vi "Analysis.Process.vi"(8 "error in (no error)":errorcluster, 11 "Parameters":T1) -> ()   [LabVIEW 2015, in "Analysis.lvlib"]
uses:
  Analysis.lvlib
  Types/Analysis.GUI.Parameters.ctl
  <vilib>/NI/AMC/Read Termination Message.vi
  <vilib>/NI/AMC/Create Single Message.vi
  <vilib>/NI/AMC/Globals.vi
  <vilib>/NI/AMC/AMC.lvlib
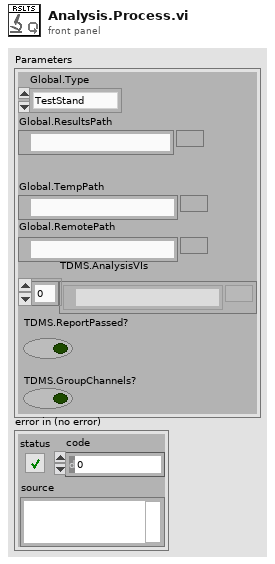
[diagram p1: front panel]
types:
  T1 = typedef "Analysis.lvlib/Analysis.GUI.Parameters.ctl" = cluster{"Global.Type":enum16{"TestStand", "TDMS"}, "Global.ResultsPath":path, "Global.TempPath":path, "Global.RemotePath":path, "TDMS.AnalysisVIs":path[], "TDMS.ReportPassed?":bool, "TDMS.GroupChannels?":bool}
  T2 = typedef "AMC.lvlib/Message Queue.ctl" = refnum<queue>
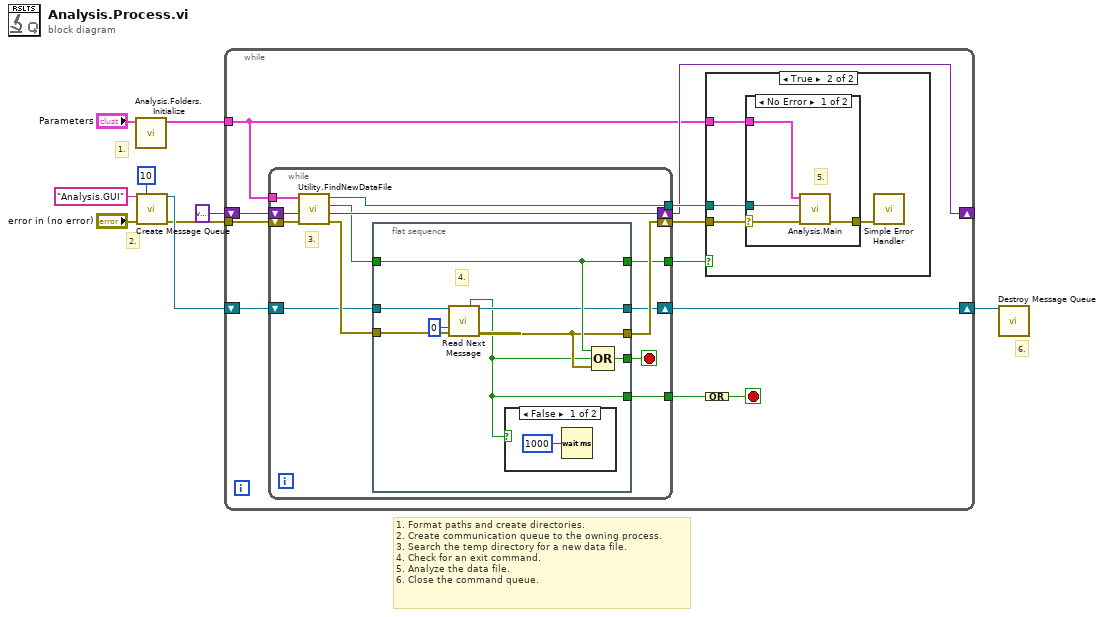
[diagram p0: block diagram]
diagram:
  # "6."
  # "1. Format paths and create directories.\n2. Create communication queue to the owning process.\n3. Search the temp directory for a new data file.\n4. Check for an exit command.\n5. Analyze the data file.\n6. Close the command queue."
  # "2."
  # "1."
  n1 = call "Analysis.Folders.Initialize.vi"("Parameters in"="Parameters") -> ("Parameters out"=w2:T1)  [unwired: 10 in]
  n2 = call <vilib>:"Create Message Queue.vi"("message queue name"="Analysis.GUI", "max queue size (-1, unlimited)"=10, "error in"="error in (no error)") -> ("message queue out"=w8:T2, "error out"=w7:errorcluster)  [unwired: 11 in]
  n3 = while {
    tunnel: w7 -> [w18]
    shift-right: [w15] -> _
    shift-left: variant -> [w16]
    tunnel: w2 -> [w12]
    shift-right: [w10] -> w9
    shift-left: w8 -> [w11]
    stop <- w19 stop-if-true
    n4 = while {
      shift-right: [w41] -> w14
      shift-left: w18 -> [w30]
      tunnel: [w34] -> w17
      tunnel: [w40] -> w13
      tunnel: [w38] -> w20
      shift-right: [w36] -> w15
      shift-left: w16 -> [w37]
      tunnel: w12 -> [w33]
      shift-right: [w31] -> w10
      shift-left: w11 -> [w32]
      stop <- w39 stop-if-true
      # "3."
      n5 = call "Utility.FindNewDataFile.vi"("error in (no error)"=w30, "LookupTable"=w37, "Parameters"=w33) -> ("error out"=w42:errorcluster, "LookupTable out"=w36:variant, "Found"=w35:bool, "Data Path"=w34:path)  [unwired: 5 in]
      n6 = flat-sequence {
        tunnel: w35 -> [w49]
        tunnel: [w50] -> w39
        tunnel: w42 -> [w47]
        tunnel: [w46] -> w41
        tunnel: [w49] -> w40
        tunnel: [w43] -> w38
        tunnel: w32 -> [w48]
        tunnel: [w44] -> w31
        frame #0 {
          # "4."
          n7 = call <vilib>:"Read Next Message.vi"("message queue in"=w48, "timeout (1 ms)"=0, "error in"=w47) -> ("exit process?"=w43:bool, "message queue out"=w44:T2, "error out"=w46:errorcluster)  [unwired: 5 in, 5 out]
          n8 = case shown="False" w43 {
            frame False {
              n9 = Wait (ms)(milliseconds to wait=u32 1000) -> ()  [unwired: 1 out]
            }
            frame True {
            }
          }
          n10 = Compound Arithmetic op=OR(w49, w43, w46) -> (w50:bool)
        }
      }
    }
    n11 = case shown="True" w13 {
      tunnel: w12 -> [_ w24]
      tunnel: w17 -> [_ w23]
      tunnel: w14 -> [_ w21]
      frame False {
      }
      frame True {
        n12 = case shown="No Error" w21 {
          selector: w21 -> [w28 w29]
          tunnel: w23 -> [w26 _]
          tunnel: w24 -> [w27 _]
          tunnel: [w25 w29] -> w22
          frame No Error {
            # "5."
            n13 = call "Analysis.Main.vi"("error in (no error)"=w28, "Data Path"=w26, "Parameters"=w27) -> ("error out"=w25:errorcluster)  [unwired: 7 in, 1 out]
          }
          frame Error {
          }
        }
        n14 = call <vilib>:"Simple Error Handler.vi"("error in (no error)"=w22) -> ()  [unwired: 4 in, 5 out]
      }
    }
    n15 = Compound Arithmetic op=OR(w20) -> (w19:bool)
  }
  n16 = call <vilib>:"Destroy Message Queue.vi"("message queue in"=w9) -> ()  [unwired: 12 in, 3 out]
